vi "Recursively Make Folders.vi"(4 "error in (no error)":errorcluster, 7 "directory path":path) -> (0 "error out":errorcluster, 3 "directory path 2":path)   [LabVIEW 2018, in "Utilities 1.lvlib"]
uses:
  Utilities 1.lvlib
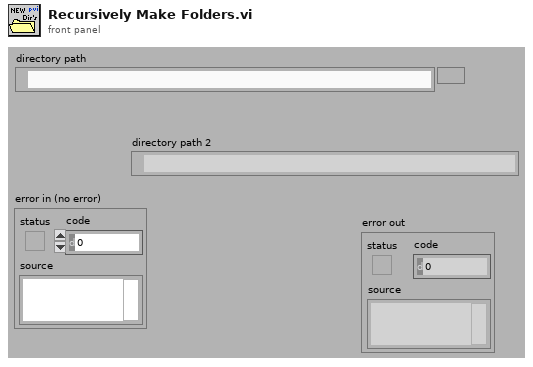
[diagram p1: front panel]
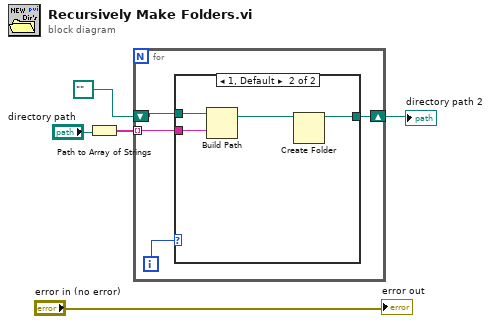
[diagram p0: block diagram]
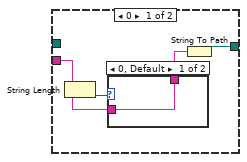
[diagram p2: hidden frame]
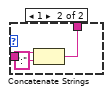
[diagram p3: hidden frame]
diagram:
  n1 = Path to Array of Strings(0:"directory path") -> (2:w4:string[])  [unwired: 1 out]
  n2 = for {
    tunnel: w4 -> [w9] mode=indexing
    shift-right: [w6] -> w2
    shift-left: path "" ("directory path") -> [w8]
    i -> [w7]
    n3 = case shown="1, Default" w7 {
      tunnel: w9 -> [w11 w20]
      tunnel: w8 -> [_ w21]
      tunnel: [w13 w18] -> w6
      frame 0 {
        n4 = String Length(string=w11) -> (length=w12:i32)
        n5 = case shown="0, Default" w12 {
          tunnel: w11 -> [w14 w17]
          tunnel: [w14 w15] -> w10
          frame 0, Default {
          }
          frame 1 {
            n6 = Concatenate Strings(w17, ":" ("string")) -> (w15:string)
          }
        }
        n7 = String To Path(string=w10) -> (path=w13:path)
      }
      frame 1, Default {
        n8 = Build Path(base path=w21, name or relative path=w20) -> (appended path=w19:path)
        n9 = Create Folder(path (use dialog)=w19) -> (created path=w18:path)  [unwired: 2 in, 2 out]
      }
    }
  }
  "directory path 2" <- w2
  "error out" <- "error in (no error)"
